vi "DAQ_AI_mean.vi"(5 "data":dbl[][](array[numeric]) format="%0.2f") -> (1 "Std":dbl[](array[numeric]), 2 "Mean":dbl[](array[numeric]))   [LabVIEW 2019]
uses:
  <vilib>/Analysis/NI_AALBase.lvlib
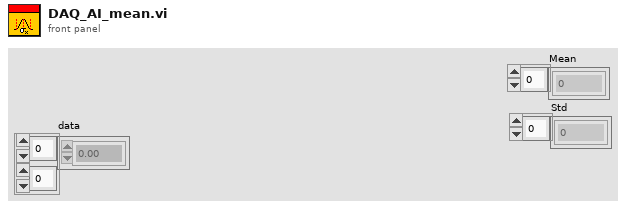
[diagram p1: front panel]
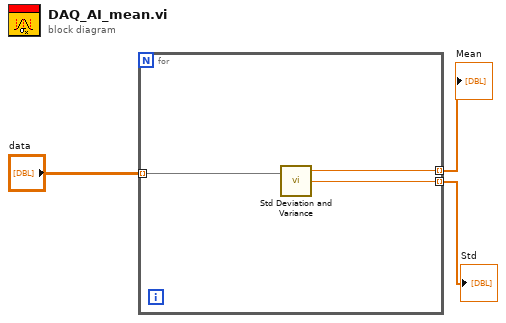
[diagram p0: block diagram]
diagram:
  n1 = for {
    tunnel: "data" -> [w6] mode=indexing
    tunnel: [w5] -> w2 mode=indexing
    tunnel: [w4] -> w1 mode=indexing
    n2 = call <vilib>:"Std Deviation and Variance.vi"("X"=w6) -> ("mean"=w5:dbl, "standard deviation"=w4:dbl)  [unwired: 1 in, 1 out]
  }
  "Mean" <- w2
  "Std" <- w1
